vi "例程06-Express频普分析.vi"() -> ()   [LabVIEW 2016]
uses:
  <vilib>/express/express analysis/Spectral/Block/exnSpectralBlock spectral measurements RMS poly.vi
  <vilib>/express/express analysis/Spectral/Block/exnSpectralBlock spectral measurements RMS DDT.vi
  <vilib>/express/express analysis/Spectral/XNode/ExpressSpectralMeasurementsBlockNode.xnode
panel:
  in  "停止":bool
  out "波形图":dynamicdata(graph)
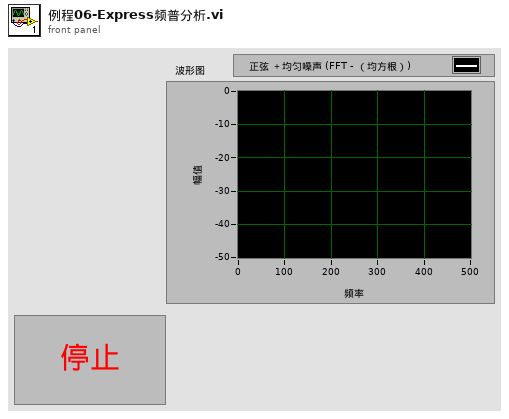
[diagram p1: front panel]
types:
  T1 = cluster{"averaging mode":u16, "weighting mode":u16, "number of averages":u32}
  T2 = cluster{"dB On (F)":bool, "unwrap phase (F)":bool, "convert to degree (F)":bool}
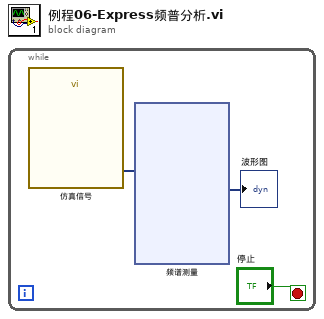
[diagram p0: block diagram]
diagram:
  n1 = while {
    stop <- "停止" stop-if-true
    n2 = call "仿真信号"() -> ("正弦与均匀噪声"=w3:dynamicdata)  [unwired: 14 in, 1 out]
    n3 = xnode "频谱测量"("信号"=w3) -> ("FFT - （均方根）"=→"波形图":dynamicdata)  [unwired: 2 in, 3 out]
  }
